vi "ChildOnly.vi"() -> (0 "error out":errorcluster)   [LabVIEW 2017, in "ResultTree.Tests.lvlib" / "AddTestCase.lvlib"]
uses:
  AddTestCase.lvlib
  ResultTree/ResultTree.lvclass
  Assertion/Assertion.lvlib
panel:
  in  "Tree":string(tree)
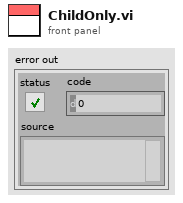
[diagram p1: front panel]
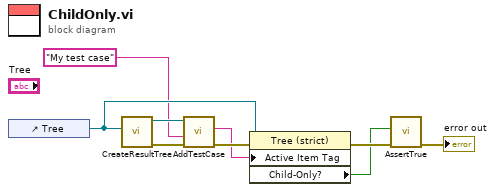
[diagram p0: block diagram]
diagram:
  n1 = control-ref of="Tree"() -> (w8:refnum<vi>)
  n2 = call "CreateResultTree.vi"("Tree Refnum"=w8) -> ("error out"=w7:errorcluster, "ResultTree out"=w5:refnum<class "ResultTree.lvclass">)  [unwired: 9 in]
  n3 = call "AddTestCase.vi"("error in (no error)"=w7, "Name"="My test case", "ResultTree in"=w5) -> ("error out"=w6:errorcluster, "Tag"=w2:string)  [unwired: 6 in, 1 out]
  n4 = property class="Tree (strict)"(reference=w8, error in=w6, "Active Item Tag"=w2) -> (error out=w4:errorcluster, "Child-Only?"=w1:bool)  [unwired: 1 out]
  n5 = call "AssertTrue.vi"("error in (no error)"=w4, "Condition"=w1) -> ("error out"=→"error out":errorcluster)  [unwired: 9 in]
